vi "rqcBob Configure Channel Test.vi"(0 "rqcBob in":refnum<class "rqcBob.lvclass">, 5 "Train.Period":u16=4000, 7 "Train.Number of Trains":u16=4000, 11 "error in (no error)":errorcluster, 12 "Window.Open":u16, 13 "Window.Close":u16=3000) -> (4 "rqcBob out":refnum<class "rqcBob.lvclass">, 15 "error out":errorcluster)   [LabVIEW 2018, in "rqcBob.lvclass"]
uses:
  rqcBob.lvclass
  Custom Controls/rqcBob Operation Mode.ctl
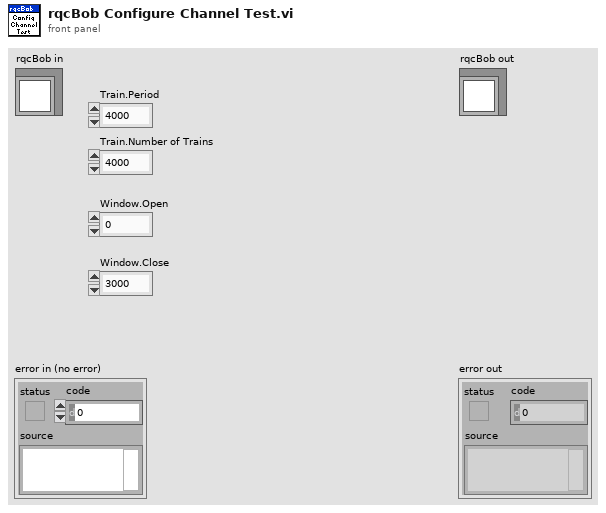
[diagram p1: front panel]
types:
  T1 = typedef "rqcBob.lvclass/rqcBob Operation Mode.ctl" = enum16{"Not Set", "Channel Test", "Key Distribution", "Modulation Level Test", "Window Test", "Delay Line Test", "Alice Modulation Level Test"}
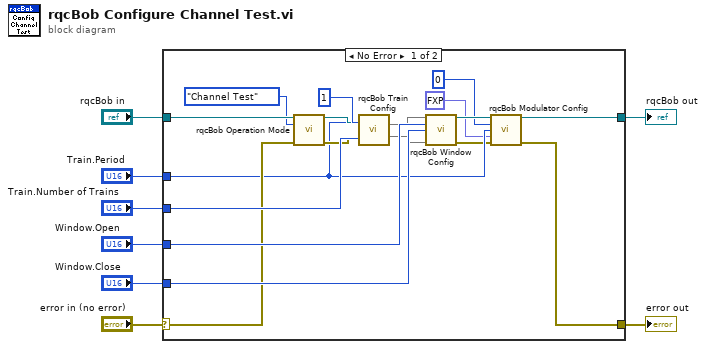
[diagram p0: block diagram]
diagram:
  n1 = case shown="No Error" "error in (no error)" {
    selector: "error in (no error)" -> [w18 w28]
    tunnel: [w9 w28] -> w7
    tunnel: [w10 w27] -> w5
    tunnel: "rqcBob in" -> [w20 w27]
    tunnel: "Train.Period" -> [w13 _]
    tunnel: "Train.Number of Trains" -> [w25 _]
    tunnel: "Window.Open" -> [w24 _]
    tunnel: "Window.Close" -> [w23 _]
    frame No Error {
      n2 = call-dynamic "rqcBob Operation Mode.vi"("rqcBob in"=w20, "Operation Mode"=rqcBob_Operation_Mode."Channel Test", "error in (no error)"=w18) -> ("rqcBob out"=w19:refnum<class "rqcBob.lvclass">, "error out"=w17:errorcluster)  [unwired: 11 in]
      n3 = call-dynamic "rqcBob Train Config.vi"("Train.Generation Mode"=w13, 2:w19, 3:u16 1 ("Number of Pulses"), "Train.First Pulse Delay Mode"=w25, "Train.First Pulse Delay"=w17) -> (6:w22, 10:w21)  [unwired: 7 in, 2 out]
      n4 = call-dynamic "rqcBob Window Config.vi"("rqcBob in"=w22, "Window.Open"=w24, "Window.Close"=w23, "error in (no error)"=w21) -> ("rqcBob out"=w15:refnum<class "rqcBob.lvclass">, "error out"=w11:errorcluster)  [unwired: 10 in]
      n5 = call-dynamic "rqcBob Modulator Config.vi"("rqcBob in"=w15, "Modulator.Start"=u16 0, "Modulator.Stop"=w13, "Modulator.Clock Delay"=fxp<+,4,4> 0.0, "error in (no error)"=w11) -> ("rqcBob out"=w10:refnum<class "rqcBob.lvclass">, "error out"=w9:errorcluster)  [unwired: 9 in]
    }
    frame Error {
    }
  }
  "error out" <- w7
  "rqcBob out" <- w5
